vi "Generic PC App.vi"() -> ()   [LabVIEW 2020]
uses:
  Volatus/Windows System SAL/Windows System SAL.lvclass
  Volatus/Volatus Core/Volatus Core.lvclass
  VolatusDAQGenericGUI/VolatusDAQGenericGUI.lvlib
  VolatusControl/VolatusControl.lvlib
  VolatusGUI/VolatusGUI.lvlib
  VolatusData/VolatusData.lvlib
  VolatusSeq/VolatusSeq.lvlib
  VolatusSeqGUI/VolatusSeqGUI.lvlib
panel:
  in  "volatus.ini path":path=path "C:/volatus/demo-app/volatus.ini"
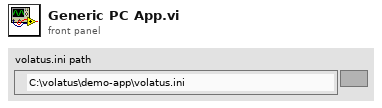
[diagram p1: front panel]
types:
  T1 = enum32{"Invalid", "Standard", "Closed", "Hidden", "Minimized", "Maximized"}
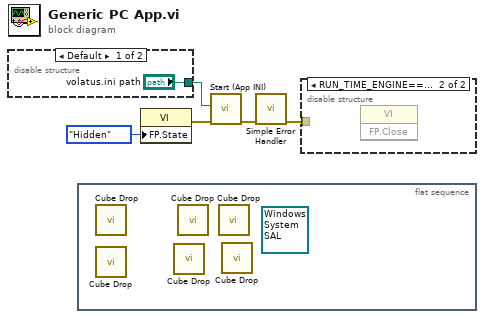
[diagram p0: block diagram]
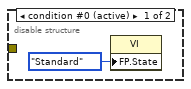
[diagram p3: hidden frame]
diagram:
  n1 = disable-structure shown="Default" {
    disable-tunnel: ["volatus.ini path" _] -> w1
    frame condition #0 (active) {
    }
    frame condition #1 {
    }
  }
  n2 = flat-sequence {
    frame #0 {
      (unwired) refnum<class "Windows System SAL.lvclass"> refnum ("Volatus:Windows System SAL.lvclass")
      n3 = call "Cube Drop.vi"() -> ()  [unwired: 12 in]
      n4 = call "Cube Drop.vi"() -> ()  [unwired: 12 in]
      n5 = call "Cube Drop.vi"() -> ()  [unwired: 12 in]
      n6 = call "Cube Drop.vi"() -> ()  [unwired: 12 in]
      n7 = call "Cube Drop.vi"() -> ()  [unwired: 12 in]
      n8 = call "Cube Drop.vi"() -> ()  [unwired: 12 in]
    }
  }
  n9 = property class="VI"("FP.State"=T1."Hidden" ("Front Panel Window:State")) -> (error out=w4:errorcluster)  [unwired: 2 in, 1 out]
  n10 = call "Start (App INI).vi"("error in (no error)"=w4, "INI Path (Default)"=w1) -> ("error out"=w5:errorcluster)  [unwired: 8 in, 1 out]
  n11 = call <vilib>:"Simple Error Handler.vi"("error in (no error)"=w5) -> ("error out"=w2:errorcluster)  [unwired: 4 in, 4 out]
  n12 = disable-structure shown="RUN_TIME_ENGINE==True" {
    disable-tunnel: w2 -> [_ _]
    frame condition #0 (active) {
      n13 = property class="VI"("FP.State"=T1."Standard" ("Front Panel Window:State")) -> ()  [unwired: 2 in, 2 out]
    }
    frame condition #1 {
      n14 = invoke class="VI" method="FP.Close"() -> ()  [unwired: 3 in, 3 out]
    }
  }
